vi "Cargo Reset.vi"(0 "Open Refnum":string, 1 "Drive Refnum":string, 2 "Outer Refnum":string, 3 "Inner Refnum":string, 4 "Other Refnum":string, 5 "Close Refnum":string, 6 "Punch Refnum":string, 7 "Ball reset?":bool) -> ()   [LabVIEW 2018]
uses:
  <vilib>/Rock Robotics/WPI/Solenoid/WPI_SolenoidValue.ctl
  <vilib>/Rock Robotics/WPI/Utilities/WPI_GetSetVariantRefNum.vi
  <vilib>/Rock Robotics/WPI/RobotDrive/WPI_RobotDriveArcadeDrive_Standard(NoSaturation).vi
  <vilib>/Rock Robotics/WPI/Solenoid/WPI_SolenoidSetEnum.vi
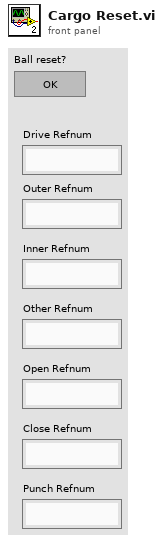
[diagram p1: front panel]
types:
  T1 = typedef "WPI_SolenoidValue.ctl" = enum16{"Off", "On", "Forward", "Reverse"}
  T2 = typedef "WPI_SolenoidDevRef.ctl" = cluster{"DevStatus":errorcluster, "Pneumatics Control Module":u8, "Forward Solenoid Channel":T3, "Reverse Solenoid Channel":T3}
  T3 = typedef "WPI_SolenoidChannel.ctl" = enum8{"Solenoid 0", "Solenoid 1", "Solenoid 2", "Solenoid 3", "Solenoid 4", "Solenoid 5", "Solenoid 6", "Solenoid 7", "Invalid"}
  T4 = typedef "WPI_RobotDriveDevRef.ctl" = cluster{"DevStatus":errorcluster, "Motors[]":T5[], "Square Inputs":bool, "Max Output":dbl}
  T5 = typedef "WPI_MotorControlDeviceRef.ctl" = cluster{"DeviceStatus":errorcluster, "Type":T6, "PWM":cluster{"PWM Channel":T7, "DeadBand":T8}, "CAN":cluster{"Device Number":u8, "SetOutput VI Ref":variant, "GetOutput VI Ref":variant, "Enable VI Ref":variant, "Disable VI Ref":variant, "Data":variant}, "Invert":bool, "DIO PWM":cluster{"PWM \"Enable\" Channel":T7, "DIOChannel":T9, "PWM Rate":dbl}}
  T6 = typedef "WPI_MotorControlType.ctl" = enum16{"PWM", "CAN", "DIO PWM"}
  T7 = typedef "FPGA_DIOPWMChannel.ctl" = enum8{"PWM 0", "PWM 1", "PWM 2", "PWM 3", "PWM 4", "PWM 5", "PWM 6", "PWM 7", "PWM 8", "PWM 9", "PWM MXP 0", "PWM MXP 1", "PWM MXP 2", "PWM MXP 3", "PWM MXP 4", "PWM MXP 5", "PWM MXP 6", "PWM MXP 7", "PWM MXP 8", "PWM MXP 9", "Invalid"}
  T8 = typedef "WPI_PWMDeadband.ctl" = cluster{"Name":string, "maxPositivePwm":i32, "minPositivePwm":i32, "centerPwm":i32, "maxNegativePwm":i32, "minNegativePwm":i32, "angularRange":u16}
  T9 = typedef "FPGA_DIOChannel.ctl" = enum8{"DIO 0", "DIO 1", "DIO 2", "DIO 3", "DIO 4", "DIO 5", "DIO 6", "DIO 7", "DIO 8", "DIO 9", "DIO MXP 0", "DIO MXP 1", "DIO MXP 2", "DIO MXP 3", "DIO MXP 4", "DIO MXP 5", "DIO MXP 6", "DIO MXP 7", "DIO MXP 8", "DIO MXP 9", "DIO MXP 10", "DIO MXP 11", "DIO MXP 12", "DIO MXP 13", "DIO MXP 14", "DIO MXP 15", "SPI Port CS1", "SPI Port CS2", "SPI Port CS3", "SPI Port MISO", "SPI Port MOSI", "Invalid"}
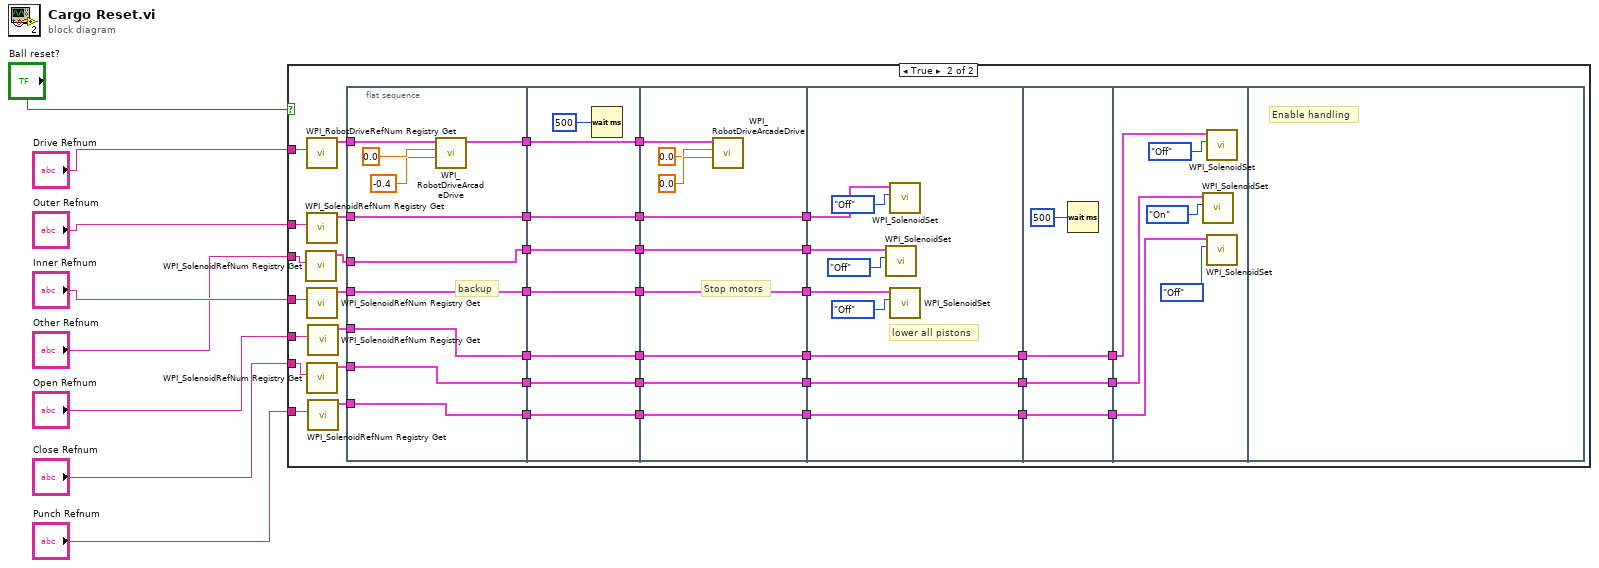
[diagram p0: block diagram]
diagram:
  n1 = case shown="True" "Ball reset?" {
    tunnel: "Drive Refnum" -> [_ w48]
    tunnel: "Outer Refnum" -> [_ w36]
    tunnel: "Inner Refnum" -> [_ w35]
    tunnel: "Other Refnum" -> [_ w30]
    tunnel: "Open Refnum" -> [_ w29]
    tunnel: "Close Refnum" -> [_ w22]
    tunnel: "Punch Refnum" -> [_ w15]
    frame False {
    }
    frame True {
      n2 = call <vilib>:"WPI_SolenoidRefNum Registry Get.vi"("refnum name"=w30) -> ("SolenoidDevRef"=w31:T2)  [unwired: 9 in, 1 out]
      n3 = call <vilib>:"WPI_RobotDriveRefNum Registry Get.vi"("refnum name"=w48) -> ("RobotDriveDevRef"=w47:T4)  [unwired: 9 in, 1 out]
      n4 = call <vilib>:"WPI_SolenoidRefNum Registry Get.vi"("refnum name"=w36) -> ("SolenoidDevRef"=w41:T2)  [unwired: 9 in, 1 out]
      n5 = call <vilib>:"WPI_SolenoidRefNum Registry Get.vi"("refnum name"=w35) -> ("SolenoidDevRef"=w37:T2)  [unwired: 9 in, 1 out]
      n6 = call <vilib>:"WPI_SolenoidRefNum Registry Get.vi"("refnum name"=w22) -> ("SolenoidDevRef"=w16:T2)  [unwired: 9 in, 1 out]
      n7 = call <vilib>:"WPI_SolenoidRefNum Registry Get.vi"("refnum name"=w29) -> ("SolenoidDevRef"=w23:T2)  [unwired: 9 in, 1 out]
      n8 = call <vilib>:"WPI_SolenoidRefNum Registry Get.vi"("refnum name"=w15) -> ("SolenoidDevRef"=w9:T2)  [unwired: 9 in, 1 out]
      n9 = flat-sequence {
        tunnel: w47 -> [w58]
        tunnel: [w55] -> w45
        tunnel: [w54] -> w42
        tunnel: w41 -> [w54]
        tunnel: [w53] -> w38
        tunnel: w37 -> [w53]
        tunnel: [w52] -> w32
        tunnel: w31 -> [w52]
        tunnel: [w51] -> w24
        tunnel: w23 -> [w51]
        tunnel: [w50] -> w17
        tunnel: w16 -> [w50]
        tunnel: [w49] -> w10
        tunnel: w9 -> [w49]
        tunnel: [w65] -> w46
        tunnel: w45 -> [w65]
        tunnel: [w64] -> w43
        tunnel: w42 -> [w64]
        tunnel: [w63] -> w39
        tunnel: w38 -> [w63]
        tunnel: [w62] -> w33
        tunnel: w32 -> [w62]
        tunnel: [w61] -> w25
        tunnel: w24 -> [w61]
        tunnel: [w60] -> w18
        tunnel: w17 -> [w60]
        tunnel: [w59] -> w11
        tunnel: w10 -> [w59]
        tunnel: w46 -> [w73]
        tunnel: [w72] -> w44
        tunnel: w43 -> [w72]
        tunnel: [w71] -> w40
        tunnel: w39 -> [w71]
        tunnel: [w70] -> w34
        tunnel: w33 -> [w70]
        tunnel: [w69] -> w26
        tunnel: w25 -> [w69]
        tunnel: [w68] -> w19
        tunnel: w18 -> [w68]
        tunnel: [w67] -> w12
        tunnel: w11 -> [w67]
        tunnel: w44 -> [w82]
        tunnel: w40 -> [w81]
        tunnel: w34 -> [w79]
        tunnel: [w78] -> w27
        tunnel: w26 -> [w78]
        tunnel: [w77] -> w20
        tunnel: w19 -> [w77]
        tunnel: [w76] -> w13
        tunnel: w12 -> [w76]
        tunnel: [w87] -> w28
        tunnel: w27 -> [w87]
        tunnel: [w86] -> w21
        tunnel: w20 -> [w86]
        tunnel: [w85] -> w14
        tunnel: w13 -> [w85]
        tunnel: w28 -> [w91]
        tunnel: w21 -> [w90]
        tunnel: w14 -> [w89]
        frame #0 {
          # "backup"
          n10 = call-poly <vilib>:"WPI_RobotDriveArcadeDrive.vi"("Y axis value"=-0.4, "X axis value"=0.0, "RobotDriveDevRef"=w58) -> ("RobotDriveDevRef"=w55:T4)  [unwired: 6 in, 2 out]
        }
        frame #1 {
          n11 = Wait (ms)(milliseconds to wait=500) -> ()  [unwired: 1 out]
        }
        frame #2 {
          # "Stop motors"
          n12 = call-poly <vilib>:"WPI_RobotDriveArcadeDrive.vi"("Y axis value"=0.0, "X axis value"=0.0, "RobotDriveDevRef"=w73) -> ()  [unwired: 6 in, 3 out]
        }
        frame #3 {
          # "lower all pistons"
          n13 = call-poly <vilib>:"WPI_SolenoidSet.vi"("Value"=WPI_SolenoidValue."Off", "SolenoidDevRef"=w79) -> ()  [unwired: 8 in, 2 out]
          n14 = call-poly <vilib>:"WPI_SolenoidSet.vi"("Value"=WPI_SolenoidValue."Off", "SolenoidDevRef"=w82) -> ()  [unwired: 8 in, 2 out]
          n15 = call-poly <vilib>:"WPI_SolenoidSet.vi"("Value"=WPI_SolenoidValue."Off", "SolenoidDevRef"=w81) -> ()  [unwired: 8 in, 2 out]
        }
        frame #4 {
          n16 = Wait (ms)(milliseconds to wait=u32 500) -> ()  [unwired: 1 out]
        }
        frame #5 {
          n17 = call-poly <vilib>:"WPI_SolenoidSet.vi"("Value"=WPI_SolenoidValue."On", "SolenoidDevRef"=w90) -> ()  [unwired: 8 in, 2 out]
          n18 = call-poly <vilib>:"WPI_SolenoidSet.vi"("Value"=WPI_SolenoidValue."Off", "SolenoidDevRef"=w91) -> ()  [unwired: 8 in, 2 out]
          n19 = call-poly <vilib>:"WPI_SolenoidSet.vi"("Value"=WPI_SolenoidValue."Off", "SolenoidDevRef"=w89) -> ()  [unwired: 8 in, 2 out]
        }
        frame #6 {
          # "Enable handling"
        }
      }
    }
  }
